vi "load_from_file.vi"() -> ()   [LabVIEW 2016]
uses:
  <vilib>/Utility/file.llb/Read Delimited Spreadsheet (DBL).vi
panel:
  in  "# hidden layers":i32=1
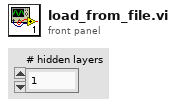
[diagram p1: front panel]
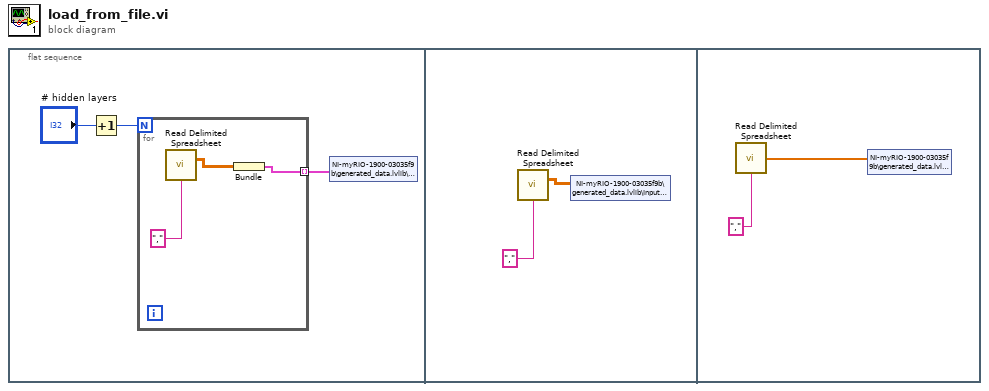
[diagram p0: block diagram]
diagram:
  n1 = flat-sequence {
    frame #0 {
      n2 = Increment(x="# hidden layers") -> (x+1=w3:i32)
      n3 = for {
        N: w3 -> [_]
        tunnel: [w4] -> w1 mode=indexing
        n4 = call-poly <vilib>:"Read Delimited Spreadsheet.vi"("delimiter (\\t)"=",") -> ("all rows"=w6:dbl[][])  [unwired: 9 in, 5 out]
        n5 = Bundle("all rows"=w6) -> (w4:cluster{"all rows":dbl[][]})  [unwired: 1 in]
      }
      n6 = shared-variable "NI-myRIO-1900-03035f9b\\generated_data.lvlib\\Weights"(w1) -> ()  [unwired: 1 in, 1 out]
    }
    frame #1 {
      n7 = call-poly <vilib>:"Read Delimited Spreadsheet.vi"("delimiter (\\t)"=",") -> ("all rows"=w7:dbl[][])  [unwired: 9 in, 5 out]
      n8 = shared-variable "NI-myRIO-1900-03035f9b\\generated_data.lvlib\\Input Data"(w7) -> ()  [unwired: 1 in, 1 out]
    }
    frame #2 {
      n9 = call-poly <vilib>:"Read Delimited Spreadsheet.vi"("delimiter (\\t)"=",") -> ("first row"=w10:dbl[])  [unwired: 9 in, 5 out]
      n10 = shared-variable "NI-myRIO-1900-03035f9b\\generated_data.lvlib\\Targets"(w10) -> ()  [unwired: 1 in, 1 out]
    }
  }
